vi "copy database to platform.vi"(11 "数据库类型":T1) -> ()   [LabVIEW 2016]
panel:
  out "error out":errorcluster
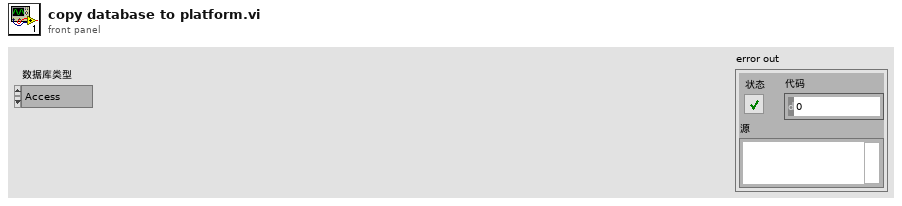
[diagram p1: front panel]
types:
  T1 = typedef "数据库类型.ctl" = enum16{"Access", "SQLite"}
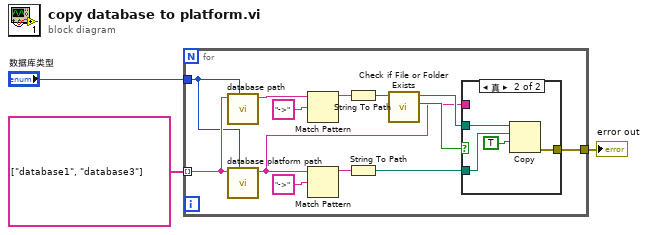
[diagram p0: block diagram]
diagram:
  n1 = for {
    tunnel: string[] ["database1", "database3"] -> [w13] mode=indexing
    tunnel: "数据库类型" -> [w12]
    tunnel: [w16] -> w1
    n2 = call "database path.vi"("数据库类型"=w12, "database"=w13) -> ("Path out"=w8:string)  [unwired: 8 in, 1 out]
    n3 = call "database platform path.vi"("数据库类型"=w12, "database"=w13) -> ("Path out"=w11:string)  [unwired: 9 in]
    n4 = Match Pattern(string=w8, regular expression="->") -> (before substring=w7:string)  [unwired: 1 in, 3 out]
    n5 = Match Pattern(string=w11, regular expression="->") -> (before substring=w6:string)  [unwired: 1 in, 3 out]
    n6 = String To Path(string=w7) -> (path=w5:path)
    n7 = String To Path(string=w6) -> (path=w4:path)
    n8 = call <vilib>:"Check if File or Folder Exists.vi"("path"=w5) -> ("file or folder exists?"=w15:bool, "dup path"=w14:path)  [unwired: 8 in, 1 out]
    n9 = case shown="真" w15 {
      tunnel: w11 -> [_ _]
      tunnel: [_ w19] -> w16
      tunnel: w14 -> [_ w18]
      tunnel: w4 -> [_ w17]
      frame False {
      }
      frame True {
        n10 = Copy(9:TRUE ("覆盖(F)"), 10:w17, 11:w18) -> (0:w19:errorcluster)  [unwired: 2 in, 2 out]
      }
    }
  }
  "error out" <- w1
